vi "terminate.vi"(8 "error in (no error)":errorcluster, 11 "WriteSignalsDAQmxPlugin in":refnum<class "SignalWriterMM140725DAQmx.lvclass">) -> (0 "error out":errorcluster, 3 "WriteSignalsDAQmxPlugin out":refnum<class "SignalWriterMM140725DAQmx.lvclass">)   [LabVIEW 2010, in "SignalWriterMM140725DAQmx.lvclass"]
uses:
  SignalWriterMM140725DAQmx.lvclass
  common/enumerations/functional_global_action_enum.ctl
  GenericSignalWriter/GenericSignalWriter/GenericSignalWriter.lvclass
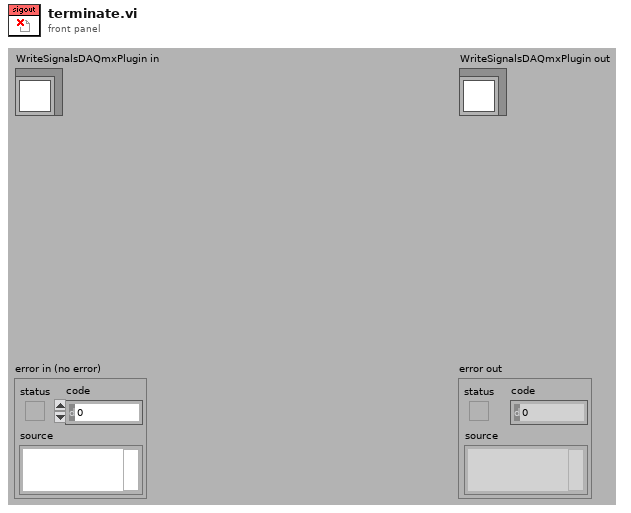
[diagram p1: front panel]
types:
  T1 = typedef "functional_global_action_enum.ctl" = enum16{"get", "set", "reset"}
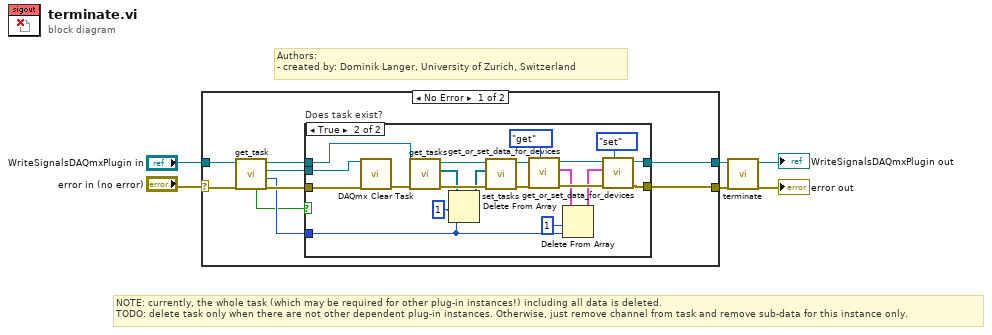
[diagram p0: block diagram]
diagram:
  # "Authors: \n- created by: Dominik Langer, University of Zurich, Switzerland"
  # "NOTE: currently, the whole task (which may be required for other plug-in instances!) including all data is deleted.\nTODO: delete task only when there are not other dependent plug-in instances. Otherwise, just remove channel from task and remove sub-data for this instance only."
  n1 = case shown="No Error" "error in (no error)" {
    selector: "error in (no error)" -> [w15 w39]
    tunnel: [w11 w39] -> w3
    tunnel: [w7 w40] -> w1
    tunnel: "WriteSignalsDAQmxPlugin in" -> [w13 w40]
    frame No Error {
      n2 = call-dynamic "get_task.vi"("error in (no error)"=w15, "DAQmxWriteSignals in"=w13) -> ("error out"=w14:errorcluster, "index"=w10:i32, "writer task"=w12:refnum<k21>, "DAQmxWriteSignals out"=w8:refnum<class "SignalWriterMM140725DAQmx.lvclass">, "found?"=w9:bool)  [unwired: 5 out]
      n3 = case "Does task exist?" shown="True" w9 {
        tunnel: w14 -> [w17 w38]
        tunnel: w12 -> [_ w37]
        tunnel: [w17 w23] -> w11
        tunnel: w10 -> [_ w19]
        tunnel: w8 -> [w16 w32]
        tunnel: [w16 w24] -> w7
        frame False {
        }
        frame True {
          n4 = call <vilib>:"DAQmx Clear Task.vi"("task in"=w37, "error in"=w38) -> ("error out"=w34:errorcluster)  [unwired: 13 out]
          n5 = call-dynamic "get_tasks.vi"("error in (no error)"=w34, "DAQmxWriteSignals in"=w32) -> ("error out"=w33:errorcluster, "output tasks"=w31:refnum<k21>[], "DAQmxWriteSignals out"=w35:refnum<class "SignalWriterMM140725DAQmx.lvclass">)  [unwired: 7 out]
          n6 = Delete From Array(array=w31, length=1, index=w19) -> (array with subset deleted=w30:refnum<k21>[])  [unwired: 1 out]
          n7 = call-dynamic "set_tasks.vi"("error in (no error)"=w33, "output tasks"=w30, "DAQmxWriteSignals in"=w35) -> ("error out"=w29:errorcluster, "DAQmxWriteSignals out"=w28:refnum<class "SignalWriterMM140725DAQmx.lvclass">)  [unwired: 1 in, 6 out]
          n8 = call-dynamic "get_or_set_data_for_devices.vi"("action"=functional_global_action_enum."get", "error in (no error)"=w29, "DAQmxWriteSignals in"=w28) -> ("error out"=w25:errorcluster, "data for devices out"=w21:cluster{"data for channels":dbl[][]}[], "DAQmxWriteSignals out"=w26:refnum<class "SignalWriterMM140725DAQmx.lvclass">)  [unwired: 1 in, 5 out]
          n9 = Delete From Array(array=w21, length=1, index=w19) -> (array with subset deleted=w20:cluster{"data for channels":dbl[][]}[])  [unwired: 1 out]
          n10 = call-dynamic "get_or_set_data_for_devices.vi"("action"=functional_global_action_enum."set", "error in (no error)"=w25, "data for devices in"=w20, "DAQmxWriteSignals in"=w26) -> ("error out"=w23:errorcluster, "DAQmxWriteSignals out"=w24:refnum<class "SignalWriterMM140725DAQmx.lvclass">)  [unwired: 6 out]
        }
      }
    }
    frame Error {
    }
  }
  n11 = call-parent "terminate.vi"("error in (no error)"=w3, "GenericPlugin in"=w1) -> ("error out"=→"error out":errorcluster, "GenericPlugin out"=→"WriteSignalsDAQmxPlugin out":refnum<class "SignalWriterMM140725DAQmx.lvclass">)  [unwired: 8 out]
